vi "Run.vi"(4 "Boolean":bool, 6 "Numeric":dbl, 7 "Database Entry in":refnum<class "Database Entry.lvclass">, 8 "error in (no error)":errorcluster, 9 "Assembly Type":string, 10 "Control In":T1={"I-O.lvclass"=refnum, "Gantry"=refnum, "Dispenser"="COM1"}, 11 "Assembly In":refnum<class "Database Assembly.lvclass">) -> (0 "error out":errorcluster, 2 "Control Out":T1={"I-O.lvclass"=refnum, "Gantry"=refnum, "Dispenser"="COM1"}, 3 "Assembly Out":refnum<class "Database Assembly.lvclass">, 5 "Database Entry out":refnum<class "Database Entry.lvclass">)   [LabVIEW 2021, in "Database Assembly.lvclass"]
uses:
  Database Assembly.lvclass
  C:/Users/HEP/Documents/GitHub/Gantry/UCSB-Gantry-HEP-main/Classes/Assembly/Assembly Run.lvclass
  Controller/Controllers.ctl
  Controller/I-O/I-O.lvclass
  C:/Program Files (x86)/Aerotech/A3200/LabVIEW/2010/Bin/Aerotech.A3200.dll
  Program Files (x86)/Aerotech/A3200/LabVIEW/2010/Bin/Aerotech.A3200.dll
  Database Entry/Database Entry.lvclass
  Database Assembly.lvclass/Database Assembly.ctl
  Assembly Run.lvclass
  Module/Module.lvclass
  Controller/Controller.lvclass
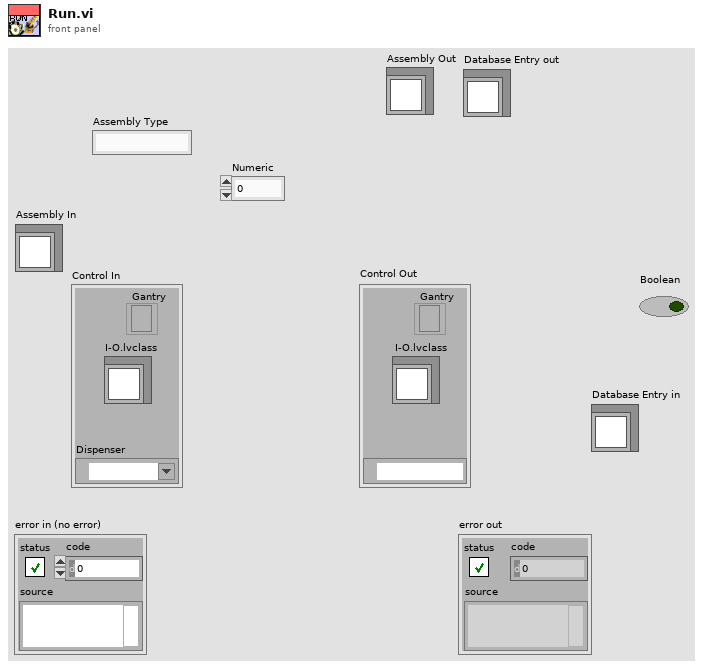
[diagram p1: front panel]
types:
  T1 = typedef "Controller.lvclass/Controllers.ctl" = cluster{"I-O.lvclass":refnum<class "I-O.lvclass">, "Gantry":refnum<k24>, "Dispenser":refnum<visa-resource-name>}
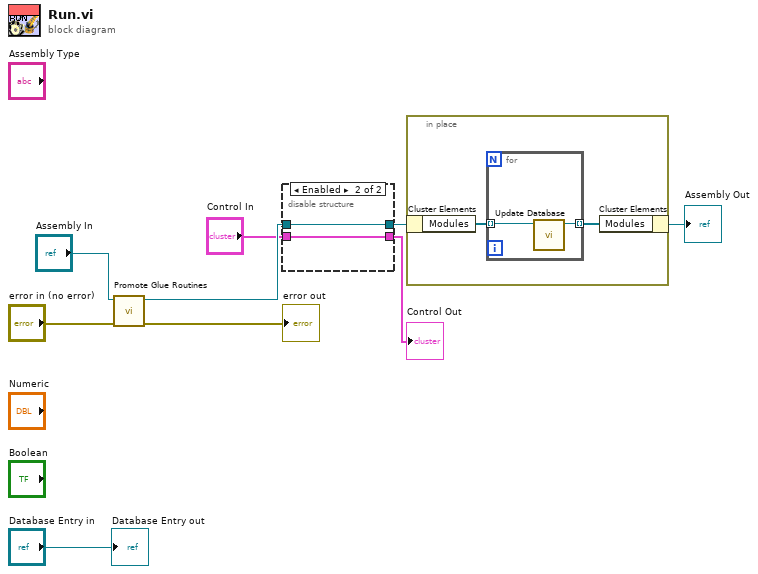
[diagram p0: block diagram]
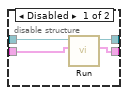
[diagram p2: hidden frame]
diagram:
  n1 = call "Promote Glue Routines.vi"("error in (no error)"="error in (no error)", "Assembly Run in"="Assembly In") -> ("error out"=→"error out":errorcluster, "Assembly Run out"=w5:refnum<class "Database Assembly.lvclass">)  [unwired: 8 in]
  n2 = disable-structure shown="Enabled" {
    disable-tunnel: w5 -> [w13 w14]
    disable-tunnel: [w12 w14] -> w4
    disable-tunnel: "Control In" -> [w11 w15]
    disable-tunnel: [w10 w15] -> w2
    frame Disabled {
      n3 = call-parent "Run.vi"("Control In"=w11, "Assembly In"=w13) -> ("Control Out"=w10:T1, "Assembly Out"=w12:refnum<class "Database Assembly.lvclass">)  [unwired: 6 in, 2 out]
    }
    frame Enabled {
    }
  }
  "Control Out" <- w2
  n4 = in-place {
    n5 = in-place-cluster #1(w4) -> ("Modules"=w17:refnum<class "Module.lvclass">[])
    n6 = for {
      tunnel: w17 -> [w19] mode=indexing
      tunnel: [w18] -> w16 mode=indexing
      n7 = call "Update Database.vi"("Module in"=w19) -> ("Module out"=w18:refnum<class "Module.lvclass">)  [unwired: 9 in, 1 out]
    }
    n8 = in-place-cluster #1("Modules"=w16) -> (→"Assembly Out":refnum<class "Database Assembly.lvclass">)
  }
  "Database Entry out" <- "Database Entry in"
